vi "Report Chamber Data.vi"(8 "error in (no error)":errorcluster, 10 "Temp (C)":dbl, 11 "Chamber Controller Interface in":refnum<class "Chamber Controller Interface.lvclass">) -> (0 "error out":errorcluster, 3 "Chamber Controller Interface out":refnum<class "Chamber Controller Interface.lvclass">)   [LabVIEW 2020, in "Chamber Controller Interfaces.lvlib" / "Chamber Controller Interface.lvclass"]
uses:
  Chamber Controller Interface.lvclass
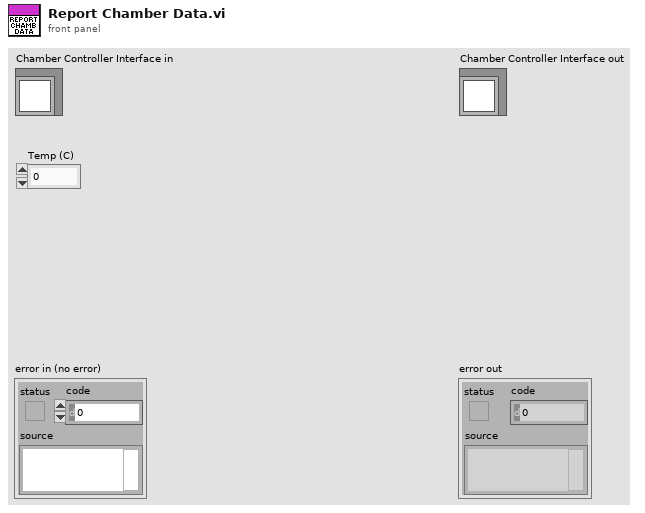
[diagram p1: front panel]
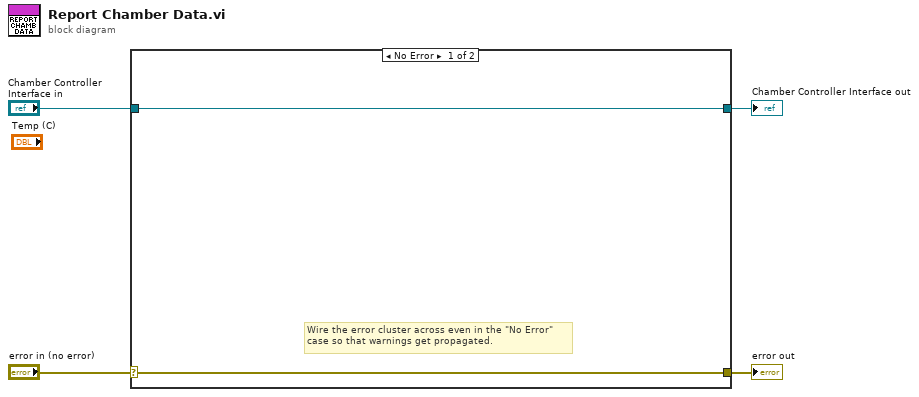
[diagram p0: block diagram]
diagram:
  n1 = case shown="No Error" "error in (no error)" {
    selector: "error in (no error)" -> [w5 w8]
    tunnel: [w5 w8] -> w3
    tunnel: [w6 w7] -> w1
    tunnel: "Chamber Controller Interface in" -> [w6 w7]
    frame No Error {
      # "Wire the error cluster across even in the \"No Error\"\ncase so that warnings get propagated."
    }
    frame Error {
    }
  }
  "error out" <- w3
  "Chamber Controller Interface out" <- w1
